vi "Load and Save Preferences.vi"() -> ()   [LabVIEW 2014]
doc: "This example shows how to use the Configuration File VIs to save key-value pairs to, and read key-value pairs from, an ini file on the robot.\n\nThis example expects a USB cable connected from your development PC to the Type B USB Jack (next to the power input) on the roboRIO."
uses:
  <vilib>/Utility/config.llb/Read Key (String).vi
  <vilib>/Utility/config.llb/Write Key (String).vi
  <vilib>/Utility/config.llb/NI_LVConfig.lvlib
panel:
  in  "Save":bool
  in  "Cancel":bool
  in  "Preferences":string[][](array[string])
  # "Use the Programming >> File I/O >> Configuration File VIs palette to save preferences on your robot across reboots or to load preferences from a file that was FTPed to the robot."
  # "Add, modify, or remove key-value pairs from this table and click save to change the contents of the preferences file."
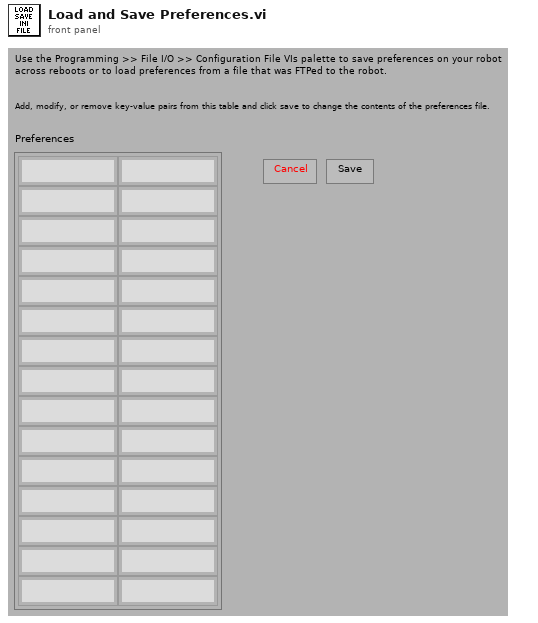
[diagram p1: front panel]
types:
  T1 = typedef "NI_LVConfig.lvlib/Config Data RefNum.ctl" = refnum<k1>
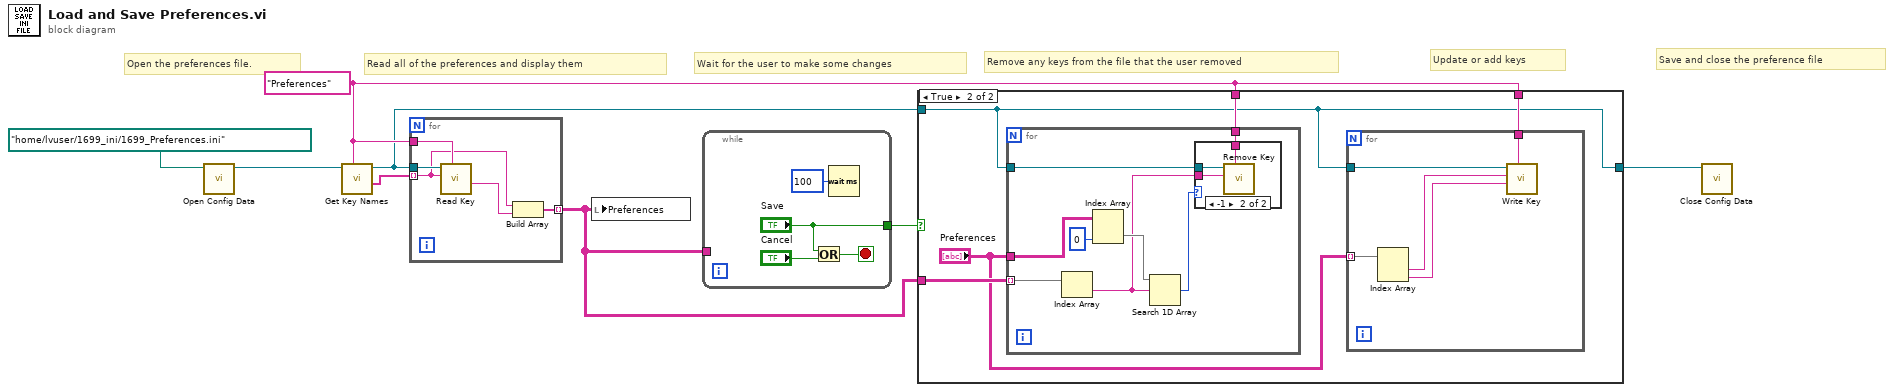
[diagram p0: block diagram]
diagram:
  w4 = "Preferences" ("section")
  # "Save and close the preference file"
  # "Update or add keys"
  # "Remove any keys from the file that the user removed"
  # "Wait for the user to make some changes"
  # "Read all of the preferences and display them"
  # "Open the preferences file."
  n1 = call <vilib>:"Open Config Data.vi"("configuration file path"=path "/home/lvuser/1699_ini/1699_Preferences.ini") -> ("refnum"=w8:T1)  [unwired: 8 in, 2 out]
  n2 = call <vilib>:"Get Key Names.vi"("section"=w4, "refnum"=w8) -> ("key names"=w7:string[], "refnum out"=w2:T1)  [unwired: 6 in, 2 out]
  n3 = for {
    tunnel: w7 -> [w11] mode=indexing
    tunnel: w2 -> [w13]
    tunnel: w4 -> [w12]
    tunnel: [w9] -> w3 mode=indexing
    n4 = call-poly <vilib>:"Read Key.vi"("section"=w12, "key"=w11, "refnum"=w13) -> ("value"=w10:string)  [unwired: 5 in, 3 out]
    n5 = Build Array(w11, w10) -> (w9:string[])
  }
  n6 = local write "Preferences"(w3) -> ()
  n7 = while {
    tunnel: ["Save"] -> w5
    tunnel: w3 -> [_]
    stop <- w16 stop-if-true
    n8 = Or(x="Save", y="Cancel") -> (x .or. y?=w16:bool)
    n9 = Wait (ms)(milliseconds to wait=u32 100) -> ()  [unwired: 1 out]
  }
  n10 = case shown="True" w5 {
    tunnel: w2 -> [w18 w20]
    tunnel: w3 -> [_ w23]
    tunnel: w4 -> [_ w22]
    tunnel: [w18 w20] -> w6
    tunnel: w4 -> [_ w21]
    frame False {
    }
    frame True {
      n11 = for {
        tunnel: w20 -> [w33]
        tunnel: w23 -> [w36] mode=indexing
        tunnel: w22 -> [w32]
        tunnel: "Preferences" -> [w29]
        n12 = Index Array(array=w36) -> (element=w31:string)  [unwired: 1 in]
        n13 = Index Array(array=w29, index (col)=0 ("disabled index (col)")) -> (element=w34:string[])  [unwired: 1 in]
        n14 = Search 1D Array(1D array=w34, element=w31) -> (index of element=w30:i32)  [unwired: 1 in]
        n15 = case shown="-1" w30 {
          tunnel: w33 -> [_ w39]
          tunnel: w32 -> [_ w38]
          tunnel: w31 -> [_ w37]
          frame 0, Default {
          }
          frame -1 {
            n16 = call <vilib>:"Remove Key.vi"("section"=w38, "key"=w37, "refnum"=w39) -> ()  [unwired: 6 in, 3 out]
          }
        }
      }
      n17 = for {
        tunnel: "Preferences" -> [w28] mode=indexing
        tunnel: w20 -> [w27]
        tunnel: w21 -> [w26]
        n18 = Index Array(array=w28) -> (element #1=w25:string, element #2=w24:string)  [unwired: 2 in]
        n19 = call-poly <vilib>:"Write Key.vi"("section"=w26, "value"=w24, "key"=w25, "refnum"=w27) -> ()  [unwired: 5 in, 3 out]
      }
    }
  }
  n20 = call <vilib>:"Close Config Data.vi"("refnum"=w6) -> ()  [unwired: 9 in, 2 out]
